vi "finder.vi"(11 "Array 3":dbl[](array[numeric])) -> (3 "Array out":i32[](array[numeric]))   [LabVIEW 2014]
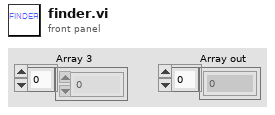
[diagram p1: front panel]
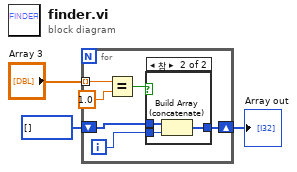
[diagram p0: block diagram]
diagram:
  n1 = for {
    tunnel: "Array 3" -> [w9] mode=indexing
    shift-right: [w5] -> w3
    shift-left: i32[] [] -> [w4]
    i -> [w6]
    n2 = Equal?(x=w9, y=1.0) -> (x = y?=w7:bool)
    n3 = case shown="참" w7 {
      tunnel: w6 -> [_ w13]
      tunnel: [w10 w12] -> w5
      tunnel: w4 -> [w10 w11]
      frame False {
      }
      frame True {
        n4 = Build Array (concatenate)(w11, w13) -> (w12:i32[])
      }
    }
  }
  "Array out" <- w3
